vi "dfd_CIC Intepolation Simu.vi"(0 "signal in":i32[](array[numeric]), 1 "lag":i32, 2 "#stage":i32, 3 "init? (T)":bool, 5 "factor":i32, 9 "Output MSB pos":i16, 11 "FXPMRateSimState in":T1, 12 "Output wl":i16, 13 "q_mode":T3=enum."Truncation" caption="rounding mode") -> (4 "signal out":i32[](array[numeric]), 15 "FXPMRateSimState out":T1)   [LabVIEW 2017, in "NI_DigFilter_FXP.lvlib"]
uses:
  <vilib>/addons/Digital Filter Design/NI_DigFilter_FXP.lvlib
  <vilib>/addons/Digital Filter Design/_Objects.llb/DFD Round-off Mode.ctl
  <vilib>/addons/Digital Filter Design/_Objects.llb/dfd_FXP MRate Simu State.ctl
  <vilib>/addons/Digital Filter Design/_Objects.llb/dfd_Integer I160.ctl
  <vilib>/addons/Digital Filter Design/NI_DigFilterLicensed.lvlib
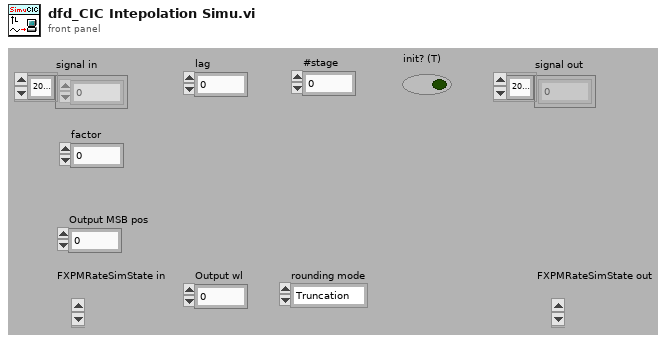
[diagram p1: front panel]
types:
  T1 = typedef "dfd_FXP MRate Simu State.ctl" = cluster{"acc1":T2[], "acc2":T2[], "FIR state":i64[], "next phase":i32}
  T2 = typedef "dfd_Integer I160.ctl" = cluster{"Hi [I32]":i32, "Lo3 [U32]":u32, "Lo2 [U32]":u32, "Lo1 [U32]":u32, "Lo0 [U32]":u32}
  T3 = typedef "NI_DigFilterLicensed.lvlib/DFD Round-off Mode.ctl" = enum16{"Nearest", "Truncation"}
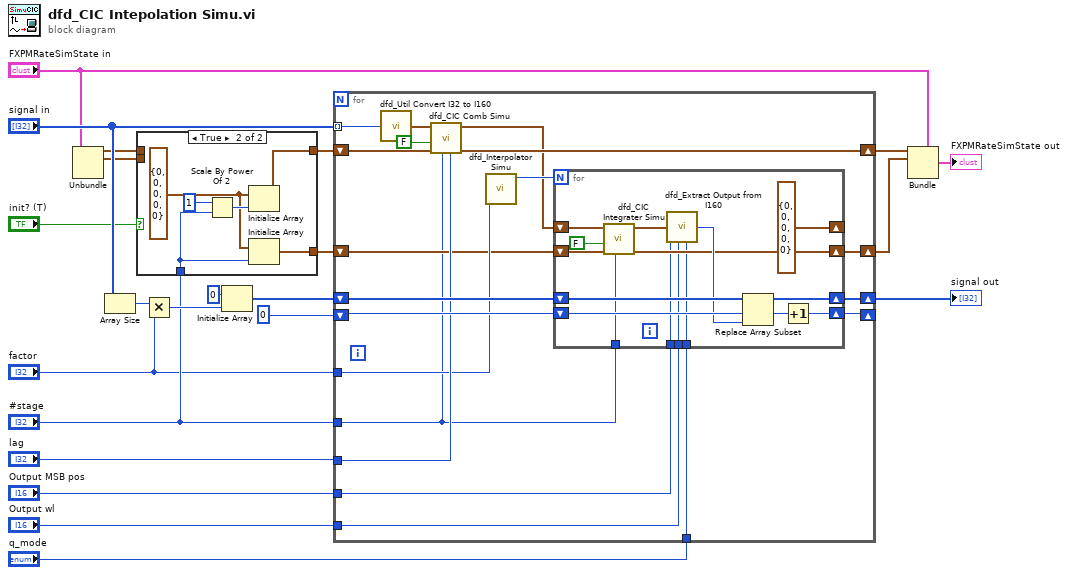
[diagram p0: block diagram]
diagram:
  n1 = Unbundle("FXPMRateSimState in") -> ("acc1"=w7:T2[], "acc2"=w6:T2[])  [unwired: 2 out]
  n2 = Array Size(array="signal in") -> (size(s)=w17:i32)
  n3 = case shown="True" "init? (T)" {
    tunnel: [w23 w27] -> w15
    tunnel: "#stage" -> [_ w26]
    tunnel: [w24 w25] -> w8
    tunnel: w7 -> [w24 _]
    tunnel: w6 -> [w23 _]
    frame False {
    }
    frame True {
      w28 = T2 {"Hi [I32]"=0, "Lo3 [U32]"=0, "Lo2 [U32]"=0, "Lo1 [U32]"=0, "Lo0 [U32]"=0} ("x [I160]")
      n4 = Scale By Power Of 2(n=1, x=w26) -> (x*2^n=w30:i32)
      n5 = Initialize Array(w28, w30) -> (w25:T2[])
      n6 = Initialize Array(w28, w26) -> (w27:T2[])
    }
  }
  n7 = Multiply(x=w17, y="factor") -> (x*y=w16:i32)
  n8 = Initialize Array(0 ("element"), w16) -> (w20:i32[])
  n9 = for {
    tunnel: "#stage" -> [w36]
    tunnel: "factor" -> [w40]
    tunnel: "signal in" -> [w45] mode=indexing
    shift-right: [w48] -> w18
    shift-left: w20 -> [w49]
    shift-right: [w46] -> _
    shift-left: 0 ("element") -> [w47]
    tunnel: "lag" -> [w41]
    shift-right: [w42] -> w5
    shift-left: w8 -> [w43]
    shift-right: [w34] -> w3
    shift-left: w15 -> [w38]
    tunnel: "Output MSB pos" -> [w35]
    tunnel: "Output wl" -> [w33]
    tunnel: "q_mode" -> [w32]
    n10 = call <vilib>:"dfd_Util Convert I32 to I160.vi"("x [I32]"=w45) -> ("x [I160]"=w44:T2)  [unwired: 8 out]
    n11 = call <vilib>:"dfd_CIC Comb Simu.vi"("lag"=w41, "#stage"=w36, "history in"=w43, "Decimation?"=FALSE, "x"=w44) -> ("history out"=w42:T2[], "y"=w37:T2)  [unwired: 1 in, 4 out]
    n12 = call <vilib>:"dfd_Interpolator Simu.vi"("factor"=w40) -> ("dup factor"=w39:i32)  [unwired: 3 in, 7 out]
    n13 = for {
      N: w39 -> [_]
      shift-right: [w62] -> w46
      shift-left: w47 -> [w63]
      shift-right: [w64] -> w48
      shift-left: w49 -> [w61]
      shift-right: [w54] -> w34
      shift-left: w38 -> [w60]
      shift-right: [T2 {"Hi [I32]"=0, "Lo3 [U32]"=0, "Lo2 [U32]"=0, "Lo1 [U32]"=0, "Lo0 [U32]"=0} ("y")] -> _
      shift-left: w37 -> [w59]
      tunnel: w36 -> [w57]
      tunnel: w35 -> [w53]
      tunnel: w33 -> [w52]
      tunnel: w32 -> [w51]
      n14 = call <vilib>:"dfd_CIC Integrater Simu.vi"("stage"=w57, "acc in"=w60, "Decimation?"=FALSE, "x"=w59) -> ("acc out"=w54:T2[], "y"=w56:T2)  [unwired: 1 in, 5 out]
      n15 = call <vilib>:"dfd_Extract Output from I160.vi"("I160"=w56, "output MSB pos"=w53, "Output wl"=w52, "q_mode"=w51) -> ("y"=w55:i32)  [unwired: 5 out]
      n16 = Replace Array Subset(array=w61, new element=w55, index=w63) -> (w64:i32[])
      n17 = Increment(x=w63) -> (x+1=w62:i32)
    }
  }
  "signal out" <- w18
  n18 = Bundle(cluster="FXPMRateSimState in", "acc1"=w5, "acc2"=w3) -> (→"FXPMRateSimState out":T1)  [unwired: 2 out]
